vi "QueueInputFile.vi"(1 "VISA resource name":refnum<visa-resource-name>, 2 "Array":string[](array[string])) -> ()   [LabVIEW 2010]
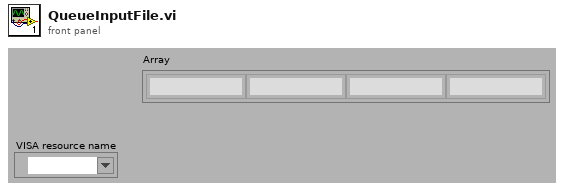
[diagram p1: front panel]
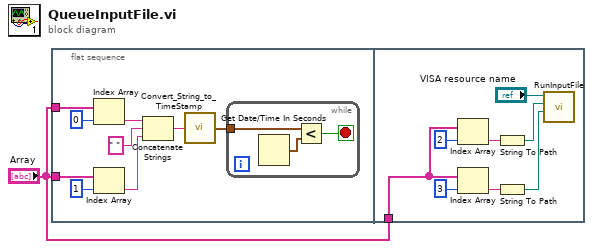
[diagram p0: block diagram]
diagram:
  n1 = flat-sequence {
    tunnel: "Array" -> [w5]
    tunnel: "Array" -> [w4]
    tunnel: "Array" -> [w17]
    frame #0 {
      n2 = Index Array(array=w5, index=0) -> (element=w9:string)
      n3 = Index Array(array=w4, index=1) -> (element=w8:string)
      n4 = Concatenate Strings(w9, " ", w8) -> (w7:string)
      n5 = call "Convert_String_to_TimeStamp.vi"("date/time string"=w7) -> ("Resulting Time Stamp"=w6:timestamp)
      n6 = while {
        tunnel: w6 -> [w13]
        stop <- w11 stop-if-true
        n7 = Get Date/Time In Seconds() -> (seconds since 1Jan1904=w12:timestamp)
        n8 = Less?(x=w13, y=w12) -> (x < y?=w11:bool)
      }
    }
    frame #1 {
      n9 = Index Array(array=w17, index=2) -> (element=w21:string)
      n10 = Index Array(array=w17, index=3) -> (element=w19:string)
      n11 = String To Path(string=w21) -> (path=w15:path)
      n12 = String To Path(string=w19) -> (path=w16:path)
      n13 = call "RunInputFile.vi"("Output Path"=w16, "Input Path"=w15, "COM Port"="VISA resource name") -> ()  [unwired: 9 in]
    }
  }
